vi "ReadAvailableRecords_5160.vi"(11 "scope params":T1={"scope mode"=enum."Stopped", "ticker"=refnum, "5160 samples per trigger"=0, "FPGA ref"=refnum, "P2P params"={"instrument handle"="", "stream session"=refnum, "scale"={"offset"=0.0, "gain"=0.0, "reserved 1"=0.0, "reserved 2"=0.0}, "actual sample rate"=10000000.0, "Trigger"=enum."PFI 0", "SCOPE Resource"="Dev1", "input impedance"=0}, "data mode"=enum."Real IO", "5782 samples per record"=0, "Chart length"=0, "RemoteConnection"=refnum, "last phase"=[]} {"P2P params"."input impedance" items=["1 mega ohm"=0, "50 ohms"=2]; "P2P params"."actual sample rate" format="%.2p"}) -> (2 "record available":bool, 3 "scope params out":T1={"scope mode"=enum."Stopped", "ticker"=refnum, "5160 samples per trigger"=0, "FPGA ref"=refnum, "P2P params"={"instrument handle"="", "stream session"=refnum, "scale"={"offset"=0.0, "gain"=0.0, "reserved 1"=0.0, "reserved 2"=0.0}, "actual sample rate"=10000000.0, "Trigger"=enum."PFI 0", "SCOPE Resource"="Dev1", "input impedance"=0}, "data mode"=enum."Real IO", "5782 samples per record"=0, "Chart length"=0, "RemoteConnection"=refnum, "last phase"=[]} {"P2P params"."input impedance" items=["1 mega ohm"=0, "50 ohms"=2]; "P2P params"."actual sample rate" format="%.2p"}, 5 "last record size 5160":u32, 7 "#elements 5160":u32)   [LabVIEW 2013]
uses:
  controls/scope_params.ctl
  Utilities/Ticker/Ticker.lvclass
  Communication/Driver/RemoteConnection/RemoteConnection.lvclass
  controls/ScopeMode.ctl
  Config/FPGAref.ctl
  P2P streaming/P2P params.ctl
  P2P streaming/trigger_source.ctl
  FPGA/DataMode.ctl
  <vilib>/rvi/interface/common/niFpgaWaitOnOcc.vi
  <vilib>/Utility/error.llb/Error Cluster From Error Code.vi
  <vilib>/rvi/errors/niLvFpgaAdjustHostInterfaceError.vi
  <vilib>/rvi/interface/nirviMethod/nirviMethod.xnode
  <vilib>/FPGAPlugInAG/Dynamic/niLvFpga_ReadFifo_Dynamic.vi
  <vilib>/rvi/errors/niLvFpgaMergeErrorWithErrorCode.vi
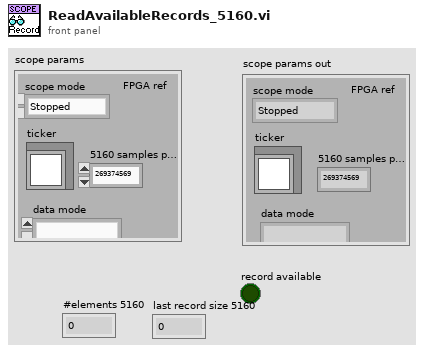
[diagram p1: front panel]
types:
  T1 = typedef "scope_params.ctl" = cluster{"scope mode":T2, "ticker":refnum<class "Ticker.lvclass">, "5160 samples per trigger":u32, "FPGA ref":T3, "P2P params":T4, "data mode":T6, "5782 samples per record":u32, "Chart length":i32, "RemoteConnection":refnum<class "RemoteConnection.lvclass">, "last phase":dbl[]}
  T2 = typedef "ScopeMode.ctl" = enum16{"Stopped", "Single", "Running", "Continuous"}
  T3 = typedef "FPGAref.ctl" = refnum<k20>
  T4 = typedef "P2P params.ctl" = cluster{"instrument handle":refnum<k15>, "stream session":refnum<k20>, "scale":cluster{"offset":dbl, "gain":dbl, "reserved 1":dbl, "reserved 2":dbl}, "actual sample rate":dbl, "Trigger":T5, "SCOPE Resource":refnum<k15>, "input impedance":u32}
  T5 = typedef "trigger_source.ctl" = enum16{"PFI 0", "PFI 1", "Software"}
  T6 = typedef "DataMode.ctl" = enum16{"Real IO", "Simulated"}
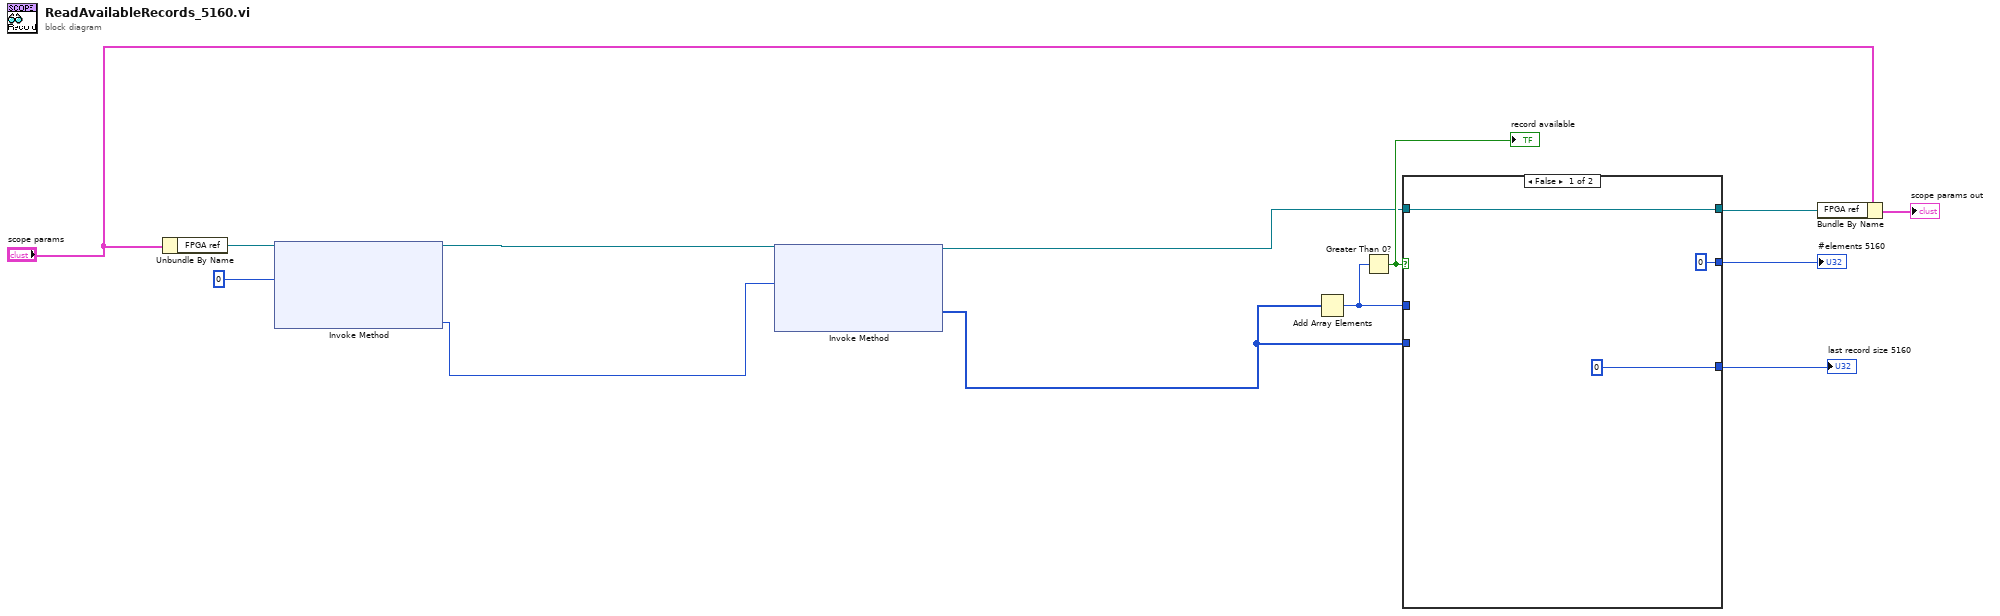
[diagram p0: block diagram]
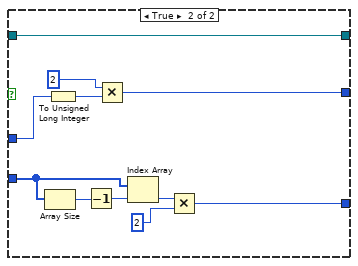
[diagram p2: hidden frame]
diagram:
  n1 = Unbundle By Name("scope params") -> ("FPGA ref"=w6:T3)
  n2 = xnode "Invoke Method"("FPGA VI Reference In"=w6, "Number of Elements"=u32 0) -> ("FPGA VI Reference Out"=w1:T3, "Elements Remaining"=w3:u32)  [unwired: 2 in, 2 out]
  n3 = xnode "Invoke Method"("FPGA VI Reference In"=w1, "Number of Elements"=w3) -> ("FPGA VI Reference Out"=w2:T3, "Data"=w4:i32[])  [unwired: 2 in, 2 out]
  n4 = Add Array Elements(numeric array=w4) -> (sum=w13:i32)
  n5 = Greater Than 0?(x=w13) -> (x > 0?=w12:bool)
  "record available" <- w12
  n6 = case shown="False" w12 {
    tunnel: w2 -> [w16 w17]
    tunnel: w13 -> [_ w24]
    tunnel: w4 -> [_ w27]
    tunnel: [w16 w17] -> w7
    tunnel: [u32 0 w19] -> w9
    tunnel: [u32 0 w18] -> w8
    frame False {
    }
    frame True {
      n7 = Array Size(array=w27) -> (size(s)=w26:i32)
      n8 = To Unsigned Long Integer(number=w24) -> (unsigned 32bit integer=w23:u32)
      n9 = Decrement(x=w26) -> (x-1=w25:i32)
      n10 = Multiply(x=u32 2, y=w23) -> (x*y=w18:u32)
      n11 = Index Array(array=w27, index=w25) -> (element=w21:i32)
      n12 = Multiply(x=w21, y=u32 2 ("x")) -> (x*y=w19:u32)
    }
  }
  "last record size 5160" <- w9
  "#elements 5160" <- w8
  n13 = Bundle By Name(cluster="scope params", "FPGA ref"=w7) -> (→"scope params out":T1)
